vi "mod_IQ Impairments DC Offset.vi"(0 "Input Complex Waveform":T1 {"Y" format="%.3f"; "dt" format="%^.2e"; "t0" format="%.4f"}, 1 "I DC Offset, %":dbl format="%.2f", 2 "Q DC Offset, %":dbl format="%.2f", 5 "Gain Scaling factor":dbl, 11 "error in (no error)":errorcluster) -> (4 "Output Complex Waveform":T1 {"Y" format="%.3f"; "dt" format="%^.2e"; "t0" format="%.4f"}, 15 "error out":errorcluster)   [LabVIEW 2020, in "niDMT.lvlib"]
doc: "Performs the DC Offset operation for IQ Impairment of an Input Data Waveform."
uses:
  <vilib>/addons/Modulation/niDMT.lvlib
  <vilib>/addons/Modulation/Analog/controls/Complex Data Waveform.ctl
  <vilib>/addons/Modulation/niAMT.lvlib
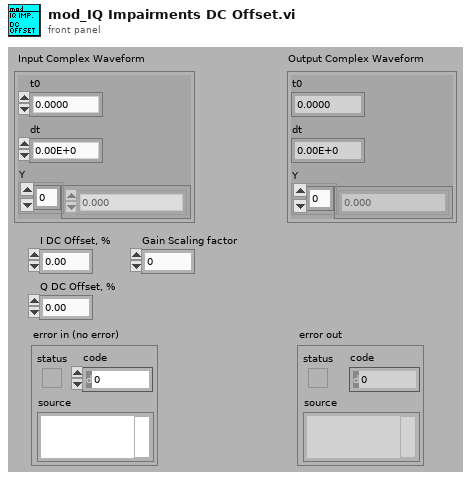
[diagram p1: front panel]
types:
  T1 = typedef "niAMT.lvlib/Complex Data Waveform.ctl" = cluster{"t0":dbl, "dt":dbl, "Y":cdb[]}
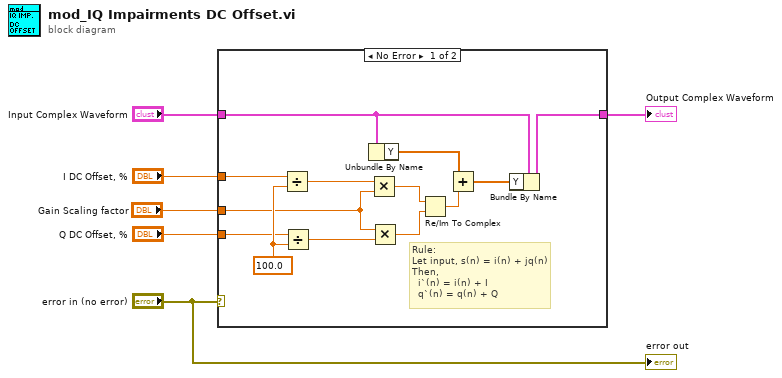
[diagram p0: block diagram]
diagram:
  n1 = case shown="No Error" "error in (no error)" {
    tunnel: "I DC Offset, %" -> [w9 _]
    tunnel: "Q DC Offset, %" -> [w8 _]
    tunnel: "Input Complex Waveform" -> [w11 w20]
    tunnel: [w10 w20] -> w3
    tunnel: "Gain Scaling factor" -> [w7 _]
    frame No Error {
      w19 = 100.0 ("y")
      # "Rule:\nLet input, s(n) = i(n) + jq(n)\nThen,\n  i`(n) = i(n) + I\n  q`(n) = q(n) + Q"
      n2 = Divide(x=w9, y=w19) -> (x/y=w17:dbl)
      n3 = Divide(x=w8, y=w19) -> (x/y=w18:dbl)
      n4 = Unbundle By Name(w11) -> ("Y"=w12:cdb[])
      n5 = Multiply(x=w17, y=w7) -> (x*y=w15:dbl)
      n6 = Multiply(x=w7, y=w18) -> (x*y=w14:dbl)
      n7 = Re/Im To Complex(1:w14, 2:w15) -> (0:w16:cdb)
      n8 = Add(x=w12, y=w16) -> (x+y=w13:cdb[])
      n9 = Bundle By Name(cluster=w11, "Y"=w13) -> (w10:T1)
    }
    frame Error {
    }
  }
  "Output Complex Waveform" <- w3
  "error out" <- "error in (no error)"
